vi "TDMS Channel Initialize.vi"(9 "Channel":string, 10 "Group":string, 11 "TDMS":string) -> (3 "TDMS Channel Info":T1)   [LabVIEW 2015]
uses:
  <userlib>/836-Library/System/TDMSv2/TDMS Channel Info.ctl
  <userlib>/836-Library/System/TDMSv2/TDMS RT FIFO Packet.ctl
  <userlib>/836-Library/System/TDMSv2/Back Channel Data.ctl
  <userlib>/836-Library/System/TDMSv2/GroupChannelIDs.ctl
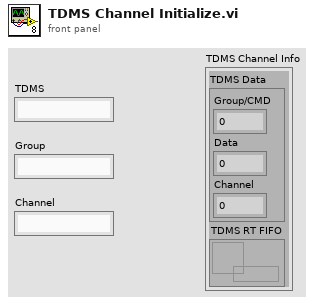
[diagram p1: front panel]
types:
  T1 = typedef "TDMS Channel Info.ctl" = cluster{"TDMS Data":T2, "TDMS RT FIFO":refnum<k33>}
  T2 = typedef "TDMS RT FIFO Packet.ctl" = cluster{"Group/CMD":i32, "Data":dbl, "Channel":i32}
  T3 = cluster{"TDMS Data":T2, "TDMS RT FIFO":refnum<k33>}
  T4 = typedef "GroupChannelIDs.ctl" = cluster{"Group":i32, "Channel":i32}
  T5 = typedef "Back Channel Data.ctl" = cluster{"Group":string, "Channel":string, "Return Notifier":refnum<notifier>}
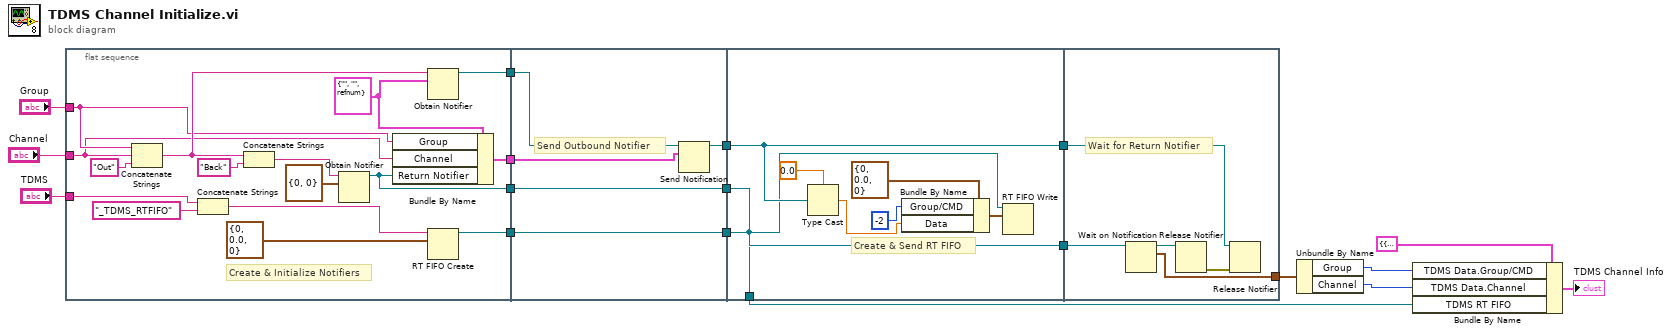
[diagram p0: block diagram]
diagram:
  n1 = flat-sequence {
    tunnel: "Group" -> [w30]
    tunnel: "Channel" -> [w29]
    tunnel: [w28] -> w18
    tunnel: [w26] -> w17
    tunnel: [w24] -> w16
    tunnel: [w23] -> w15
    tunnel: "TDMS" -> [w21]
    tunnel: w18 -> [w39]
    tunnel: [w38] -> w14
    tunnel: w17 -> [w38]
    tunnel: [w37] -> w13
    tunnel: w16 -> [w36]
    tunnel: [w35] -> w12
    tunnel: w15 -> [w35]
    tunnel: [w46] -> w11
    tunnel: w14 -> [w46]
    tunnel: [w45] -> w10
    tunnel: w13 -> [w45]
    tunnel: w12 -> [w40]
    tunnel: [w40] -> w2
    tunnel: w11 -> [w52]
    tunnel: w10 -> [w49]
    tunnel: [w48] -> w6
    frame #0 {
      w25 = T5 {"Group"="", "Channel"="", "Return Notifier"=refnum}
      # "Create & Initialize Notifiers"
      n2 = Concatenate Strings(w30, w29, "Out" ("string")) -> (w34:string)
      n3 = Concatenate Strings(w21, "_TDMS_RTFIFO" ("string")) -> (w20:string)
      n4 = Concatenate Strings(w34, "Back" ("string")) -> (w33:string)
      n5 = Obtain Notifier(name (unnamed)=w33, notification data type=T4 {"Group"=0, "Channel"=0}) -> (notifier out=w26:refnum<notifier>)  [unwired: 2 in, 2 out]
      n6 = Bundle By Name(cluster=w25, "Group"=w30, "Channel"=w29, "Return Notifier"=w26) -> (w24:T5)
      n7 = Obtain Notifier(name (unnamed)=w34, notification data type=w25) -> (notifier out=w28:refnum<notifier>)  [unwired: 2 in, 2 out]
      n8 = RT FIFO Create(0:w20, 1:T2 {"Group/CMD"=0, "Data"=0.0, "Channel"=0}) -> (8:w23:refnum<k33>)  [unwired: 6 in, 2 out]
    }
    frame #1 {
      # "Send Outbound Notifier"
      n9 = Send Notification(notification=w36, notifier=w39) -> (notifier out=w37:refnum<notifier>)  [unwired: 1 in, 1 out]
    }
    frame #2 {
      # "Create & Send RT FIFO"
      n10 = Type Cast(type=0.0, x=w45) -> (*(type *) &x=w43:dbl)
      n11 = Bundle By Name(cluster=T2 {"Group/CMD"=0, "Data"=0.0, "Channel"=0}, "Group/CMD"=-2, "Data"=w43) -> (w41:T2)
      n12 = RT FIFO Write(0:w40, 1:w41) -> ()  [unwired: 3 in, 4 out]
    }
    frame #3 {
      # "Wait for Return Notifier"
      n13 = Wait on Notification(notifier=w52) -> (notifier out=w51:refnum<notifier>, notification=w48:T4)  [unwired: 3 in, 2 out]
      n14 = Release Notifier(notifier=w51) -> (error out=w50:errorcluster)  [unwired: 2 in, 2 out]
      n15 = Release Notifier(notifier=w49, error in (no error)=w50) -> ()  [unwired: 1 in, 3 out]
    }
  }
  n16 = Unbundle By Name(w6) -> ("Group"=w5:i32, "Channel"=w4:i32)
  n17 = Bundle By Name(cluster=T3 {"TDMS Data"={"Group/CMD"=0, "Data"=0.0, "Channel"=0}, "TDMS RT FIFO"=refnum}, "TDMS Data.Group/CMD"=w5, "TDMS Data.Channel"=w4, "TDMS RT FIFO"=w2) -> (→"TDMS Channel Info":T3)
